vi "Prepend to Log.vi"(10 "new entry":string) -> (11 "Log out":string)   [LabVIEW 2023]
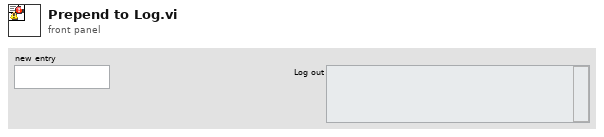
[diagram p1: front panel]
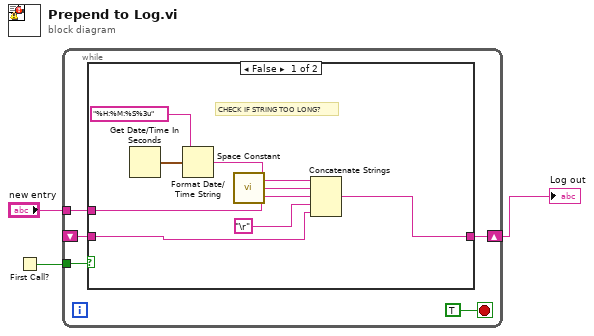
[diagram p0: block diagram]
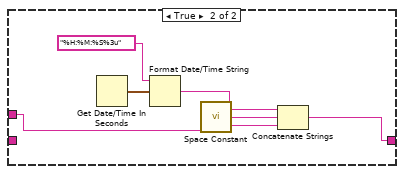
[diagram p2: hidden frame]
diagram:
  n1 = First Call?() -> (First Call?: T/F=w1:bool)
  n2 = while {
    tunnel: "new entry" -> [w7]
    shift-right: [w6] -> w3
    shift-left: _ -> [w5]
    tunnel: w1 -> [w4]
    stop <- TRUE stop-if-true
    n3 = case shown="False" w4 {
      tunnel: w7 -> [w11 w19]
      tunnel: [w10 w17] -> w6
      tunnel: w5 -> [w9 _]
      frame False {
        # "CHECK IF STRING TOO LONG?"
        n4 = Get Date/Time In Seconds() -> (seconds since 1Jan1904=w16:timestamp)
        n5 = Format Date/Time String(time format string (%c)="%H:%M:%S%3u", seconds (now)=w16) -> (date/time string=w13:string)  [unwired: 1 in]
        n6 = call <vilib>:"Space Constant.vi"() -> ("String"=w14:string)
        n7 = Concatenate Strings(w13, w14, w11, "\r", w9) -> (w10:string)
      }
      frame True {
        n8 = Get Date/Time In Seconds() -> (seconds since 1Jan1904=w22:timestamp)
        n9 = Format Date/Time String(time format string (%c)="%H:%M:%S%3u", seconds (now)=w22) -> (date/time string=w20:string)  [unwired: 1 in]
        n10 = call <vilib>:"Space Constant.vi"() -> ("String"=w21:string)
        n11 = Concatenate Strings(w20, w21, w19) -> (w17:string)
      }
    }
  }
  "Log out" <- w3
